vi "Write AO Value.vi"(8 "error in (no error)":errorcluster, 9 "AO In":dbl[](array[numeric]), 11 "PXIe 6363 in":refnum<class "PXIe 6363.lvclass">) -> (0 "error out":errorcluster, 3 "PXIe 6363 out":refnum<class "PXIe 6363.lvclass">)   [LabVIEW 2021, in "DAQ Hardware.lvlib" / "PXIe 6363.lvclass"]
uses:
  PXIe 6363.lvclass
  PXIe 6363.lvclass/PXIe 6363.ctl
  <vilib>/DAQmx/write.llb/DAQmx Write (Analog 1D DBL NChan 1Samp).vi
  <vilib>/DAQmx/miscellaneous.llb/DAQmx Fill In Error Info.vi
panel:
  out "AO 2":dbl[](array[numeric])
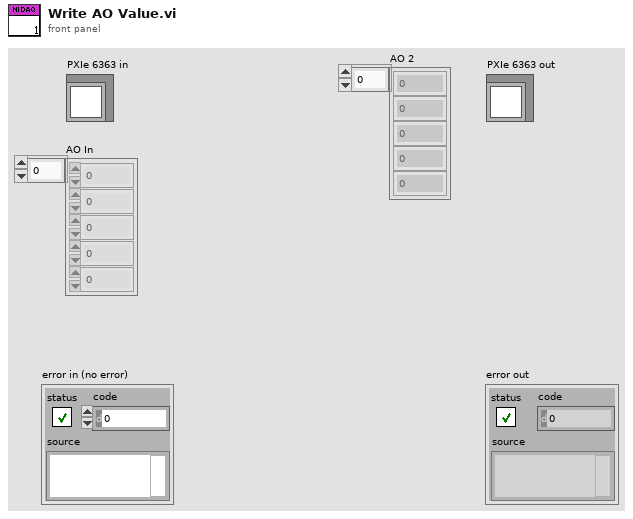
[diagram p1: front panel]
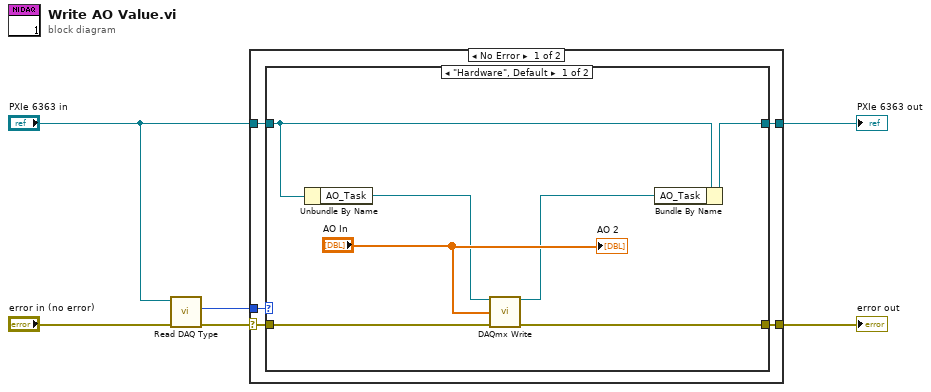
[diagram p0: block diagram]
diagram:
  n1 = call-dynamic "Read DAQ Type.vi"("error in (no error)"="error in (no error)", "PXIe 6363 in"="PXIe 6363 in") -> ("error out"=w5:errorcluster, "DAQ Type"=w4:enum16{"Hardware", "Simulation"})  [unwired: 7 in, 1 out]
  n2 = case shown="No Error" w5 {
    selector: w5 -> [w11 w21]
    tunnel: w4 -> [w10 _]
    tunnel: "PXIe 6363 in" -> [w9 w22]
    tunnel: [w8 w22] -> w2
    tunnel: [w7 w21] -> w1
    frame No Error {
      n3 = case shown="\"Hardware\", Default" w10 {
        tunnel: w11 -> [w18 w19]
        tunnel: w9 -> [w16 w20]
        tunnel: [w14 w20] -> w8
        tunnel: [w15 w19] -> w7
        frame "Hardware", Default {
          n4 = Unbundle By Name(w16) -> ("AO_Task"=w13:refnum<k21>)
          n5 = call-poly <vilib>:"DAQmx Write.vi"("task/channels in"=w13, "data"="AO In", "error in"=w18) -> ("task out"=w12:refnum<k21>, "error out"=w15:errorcluster)  [unwired: 10 in, 1 out]
          n6 = Bundle By Name(cluster=w16, "AO_Task"=w12) -> (w14:refnum<class "PXIe 6363.lvclass">)
          "AO 2" <- "AO In"
        }
        frame "Simulation" {
        }
      }
    }
    frame Error {
    }
  }
  "error out" <- w1
  "PXIe 6363 out" <- w2
